vi "lfield_set_roi.vi"(8 "error in (no error)":errorcluster, 11 "lightfield_class in":refnum<class "lightfield_class.lvclass">) -> (0 "error out":errorcluster, 3 "lightfield_class out":refnum<class "lightfield_class.lvclass">)   [LabVIEW 2015, in "lightfield_class.lvclass"]
uses:
  lightfield_class.lvclass
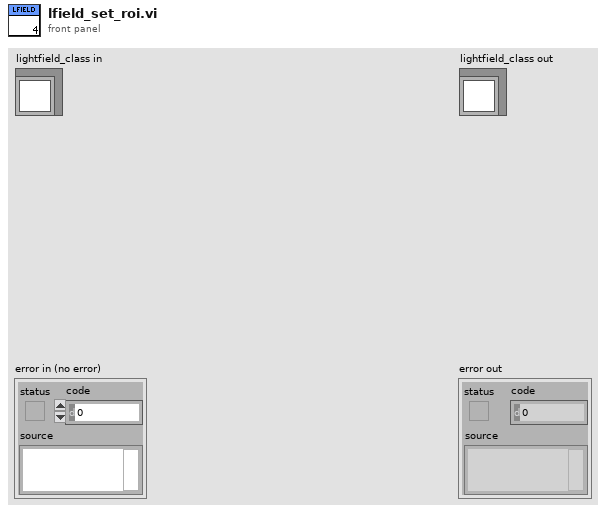
[diagram p1: front panel]
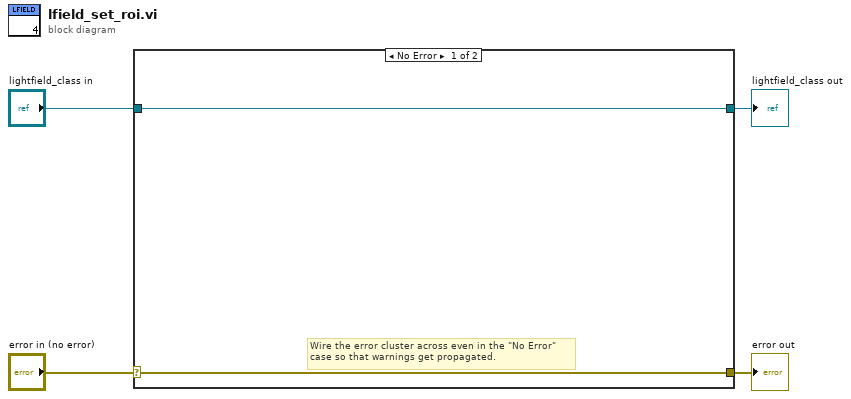
[diagram p0: block diagram]
diagram:
  n1 = case shown="No Error" "error in (no error)" {
    selector: "error in (no error)" -> [w5 w8]
    tunnel: [w5 w8] -> w3
    tunnel: [w6 w7] -> w1
    tunnel: "lightfield_class in" -> [w6 w7]
    frame No Error {
      # "Wire the error cluster across even in the \"No Error\"\ncase so that warnings get propagated."
    }
    frame Error {
    }
  }
  "error out" <- w3
  "lightfield_class out" <- w1
